vi "Evaluate.vi"(9 "Variable Values":dbl[](array[numeric]), 10 "Values":dbl[](array[numeric]), 11 "Types":T1[](array[typedef])) -> (3 "Evalulated":dbl)   [LabVIEW 2022 SP3, in "Interlocks.lvlib"]
uses:
  Interlocks.lvlib
  Controls/Token Type.ctl
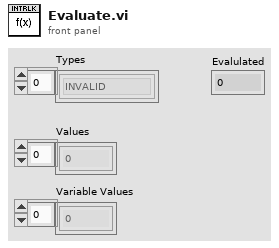
[diagram p1: front panel]
types:
  T1 = typedef "Interlocks.lvlib/Token Type.ctl" = enum8{"INVALID", "NOT", "AND", "OR", "EE", "NE", "LT", "GT", "LTE", "GTE", "PLUS", "MINUS", "MULTIPLY", "DIVIDE", "MODULUS", "LPAREN", "RPAREN", "LITERAL", "IDENTIFIER", "DEFINITION"}
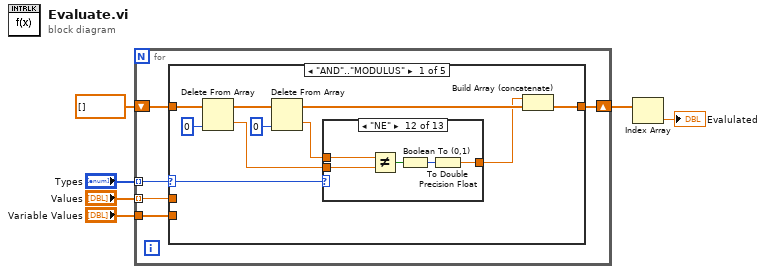
[diagram p0: block diagram]
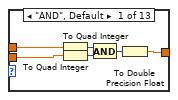
[diagram p2: hidden frame]
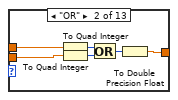
[diagram p3: hidden frame]
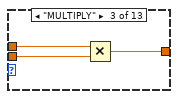
[diagram p4: hidden frame]
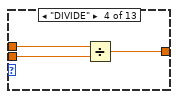
[diagram p5: hidden frame]
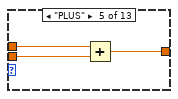
[diagram p6: hidden frame]
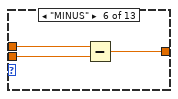
[diagram p7: hidden frame]
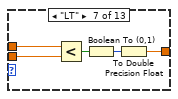
[diagram p8: hidden frame]
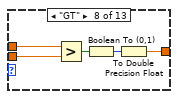
[diagram p9: hidden frame]
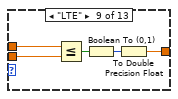
[diagram p10: hidden frame]
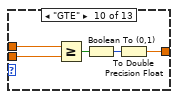
[diagram p11: hidden frame]
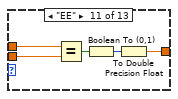
[diagram p12: hidden frame]
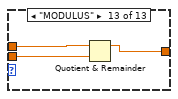
[diagram p13: hidden frame]
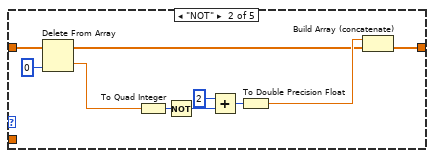
[diagram p14: hidden frame]
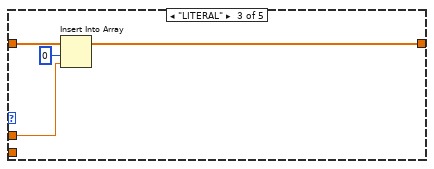
[diagram p15: hidden frame]
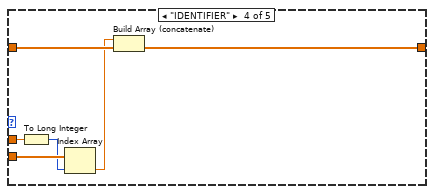
[diagram p16: hidden frame]
diagram:
  n1 = for {
    shift-right: [w11] -> w4
    shift-left: dbl[] [] -> [w10]
    tunnel: "Variable Values" -> [w9]
    tunnel: "Types" -> [w8] mode=indexing
    tunnel: "Values" -> [w7] mode=indexing
    n2 = case shown="\"AND\"..\"MODULUS\"" w8 {
      selector: w8 -> [w12 _ _ _ _]
      tunnel: w7 -> [_ _ w89 w94 _]
      tunnel: [w17 w86 w92 w95 w99] -> w11
      tunnel: w10 -> [w21 w88 w91 w97 w99]
      tunnel: w9 -> [_ _ _ w98 _]
      frame "AND".."MODULUS" {
        n3 = Delete From Array(array=w21, index=0) -> (deleted portion=w16:dbl, array with subset deleted=w19:dbl[])  [unwired: 1 in]
        n4 = Delete From Array(array=w19, index=0) -> (deleted portion=w13:dbl, array with subset deleted=w18:dbl[])  [unwired: 1 in]
        n5 = case shown="\"NE\"" w12 {
          tunnel: w16 -> [w27 w33 w35 w38 w41 w44 w49 w54 w59 w64 w69 w74 w77]
          tunnel: [w26 w32 w34 w37 w40 w43 w46 w51 w56 w61 w66 w71 w76] -> w15
          tunnel: w13 -> [w25 w31 w36 w39 w42 w45 w50 w55 w60 w65 w70 w75 w78]
          frame "AND", Default {
            n6 = To Quad Integer(1:w25) -> (0:w23:i64)
            n7 = To Quad Integer(1:w27) -> (0:w24:i64)
            n8 = And(x=w23, y=w24) -> (x .and. y?=w22:i64)
            n9 = To Double Precision Float(number=w22) -> (double precision float=w26:dbl)
          }
          frame "OR" {
            n10 = To Quad Integer(1:w31) -> (0:w29:i64)
            n11 = To Quad Integer(1:w33) -> (0:w30:i64)
            n12 = Or(x=w29, y=w30) -> (x .or. y?=w28:i64)
            n13 = To Double Precision Float(number=w28) -> (double precision float=w32:dbl)
          }
          frame "MULTIPLY" {
            n14 = Multiply(x=w36, y=w35) -> (x*y=w34:dbl)
          }
          frame "DIVIDE" {
            n15 = Divide(x=w39, y=w38) -> (x/y=w37:dbl)
          }
          frame "PLUS" {
            n16 = Add(x=w42, y=w41) -> (x+y=w40:dbl)
          }
          frame "MINUS" {
            n17 = Subtract(x=w45, y=w44) -> (x-y=w43:dbl)
          }
          frame "LT" {
            n18 = Less?(x=w50, y=w49) -> (x < y?=w48:bool)
            n19 = Boolean To (0,1)(Boolean=w48) -> (0, 1=w47:i16)
            n20 = To Double Precision Float(number=w47) -> (double precision float=w46:dbl)
          }
          frame "GT" {
            n21 = Greater?(x=w55, y=w54) -> (0:w53:bool)
            n22 = Boolean To (0,1)(Boolean=w53) -> (0, 1=w52:i16)
            n23 = To Double Precision Float(number=w52) -> (double precision float=w51:dbl)
          }
          frame "LTE" {
            n24 = Less Or Equal?(x=w60, y=w59) -> (x <= y?=w58:bool)
            n25 = Boolean To (0,1)(Boolean=w58) -> (0, 1=w57:i16)
            n26 = To Double Precision Float(number=w57) -> (double precision float=w56:dbl)
          }
          frame "GTE" {
            n27 = Greater Or Equal?(x=w65, y=w64) -> (x >= y?=w63:bool)
            n28 = Boolean To (0,1)(Boolean=w63) -> (0, 1=w62:i16)
            n29 = To Double Precision Float(number=w62) -> (double precision float=w61:dbl)
          }
          frame "EE" {
            n30 = Equal?(x=w70, y=w69) -> (x = y?=w68:bool)
            n31 = Boolean To (0,1)(Boolean=w68) -> (0, 1=w67:i16)
            n32 = To Double Precision Float(number=w67) -> (double precision float=w66:dbl)
          }
          frame "NE" {
            n33 = Not Equal?(x=w75, y=w74) -> (x != y?=w73:bool)
            n34 = Boolean To (0,1)(Boolean=w73) -> (0, 1=w72:i16)
            n35 = To Double Precision Float(number=w72) -> (double precision float=w71:dbl)
          }
          frame "MODULUS" {
            n36 = Quotient & Remainder(x=w78, y=w77) -> (x-y*floor(x/y)=w76:dbl)  [unwired: 1 out]
          }
        }
        n37 = Build Array (concatenate)(w15, w18) -> (w17:dbl[])
      }
      frame "NOT" {
        n38 = Delete From Array(array=w88, index=0) -> (deleted portion=w85:dbl, array with subset deleted=w83:dbl[])  [unwired: 1 in]
        n39 = To Quad Integer(1:w85) -> (0:w82:i64)
        n40 = Not(x=w82) -> (.not. x?=w81:i64)
        n41 = Add(x=i64 2, y=w81) -> (x+y=w79:i64)
        n42 = To Double Precision Float(number=w79) -> (double precision float=w84:dbl)
        n43 = Build Array (concatenate)(w84, w83) -> (w86:dbl[])
      }
      frame "LITERAL" {
        n44 = Insert Into Array(array=w91, index=0, new element=w89) -> (w92:dbl[])
      }
      frame "IDENTIFIER" {
        n45 = To Long Integer(number=w94) -> (32bit integer=w93:i32)
        n46 = Index Array(array=w98, index=w93) -> (element=w96:dbl)
        n47 = Build Array (concatenate)(w96, w97) -> (w95:dbl[])
      }
      frame "INVALID", "LPAREN", "RPAREN", "DEFINITION" {
      }
    }
  }
  n48 = Index Array(array=w4) -> (element=→"Evalulated":dbl)  [unwired: 1 in]
